vi "Convert Point 2D (SGL) to Point 2D (I32).vi"(11 "Point 2D (Float)":T2) -> (3 "Point 2D (I32)":T1)   [LabVIEW 2020, in "3D (FPGA).lvlib"]
uses:
  3D (FPGA).lvlib
  Point 2D (SGL).ctl
  Raster/Point 2D (I32).ctl
  Raster/Raster (FPGA).lvlib
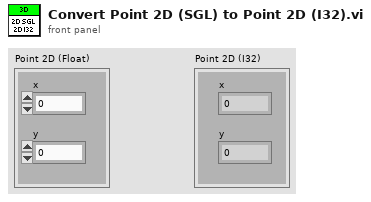
[diagram p1: front panel]
types:
  T1 = typedef "Raster (FPGA).lvlib/Point 2D (I32).ctl" = cluster{"x":i32, "y":i32}
  T2 = typedef "3D (FPGA).lvlib/Point 2D (SGL).ctl" = cluster{"x":sgl, "y":sgl}
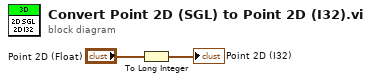
[diagram p0: block diagram]
diagram:
  n1 = To Long Integer(number="Point 2D (Float)") -> (32bit integer=→"Point 2D (I32)":cluster{"x":i32, "y":i32})
